vi "Compare Ch with Ch List.vi"(8 "error in (no error)":errorcluster, 10 "Compare List":refnum<class "ChannelVS.lvclass">[](array[class]), 11 "Channel to compare":refnum<class "ChannelVS.lvclass">) -> (0 "error out":errorcluster, 3 "Channel out":refnum<class "ChannelVS.lvclass">)   [LabVIEW 2020, in "Shared Variables CD 2.0 Configuration.lvlib" / "ChannelVS.lvclass"]
uses:
  ChannelVS.lvclass
  ChannelVS.lvclass/ChannelVS.ctl
  built/windows/Channel.lvlibp/Channel.lvclass
  built/windows/Channel.lvlibp/1abvi3w/vi.lib/Utility/Data Type/Type Definitions/Data Type.ctl
  built/windows/Channel.lvlibp/1abvi3w/vi.lib/Utility/Data Type/NI_Data Type.lvlib
  <vilib>/NI VeriStand/Custom Device API/Custom Device Item Ref.ctl
  <vilib>/NI VeriStand/Custom Device API/Custom Device API.lvlib
  C:/Users/Administrator/Desktop/GIT/Shared-Variable-Custom-Device-2.0/Source/built/windows/Channel.lvlibp/Channel.lvclass
  C:/Users/Administrator/Desktop/GIT/Shared-Variable-Custom-Device-2.0/Source/Shared Variables CD 2.0/Configuration/Support/ChannelVS/ChannelVS.lvclass
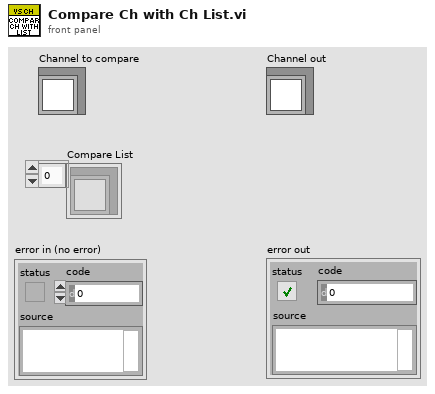
[diagram p1: front panel]
types:
  T1 = typedef "Custom Device API.lvlib/Custom Device Item Ref.ctl" = u64
  T2 = typedef "Channel.lvlibp/NI_Data Type.lvlib/Data Type.ctl" = enum8{"Invalid Type", "Void", "I8", "I16", "I32", "I64", "U8", "U16", "U32", "U64", "Single Float", "Double Float", "Extended Float", "Single Complex", "Double Complex", "Extended Complex", "Enum U8", "Enum U16", "Enum U32", "Enum U64", "Single Float With Unit", "Double Float With Unit", "Extended Float With Unit", "Single Complex with Unit", "Double Complex with Unit", "Extended Complex with Unit", "Boolean", "String", "Path", "Picture", "Tag", "Array", "Cluster", "Variant", "LV Variant", "Waveform", "Timestamp", "Digital Waveform", "Digital Data", "ExpressData", "Refnum", "External Data", "VI", "Poly VI", "LabVIEW Class Instance", "Fixed Point", "Set Collection", "Map Collection"}
  T3 = cluster{"Name":string, "URL":string, "DataType":T2}
  T4 = cluster{"Name":bool, "URL":bool, "DataType":bool}
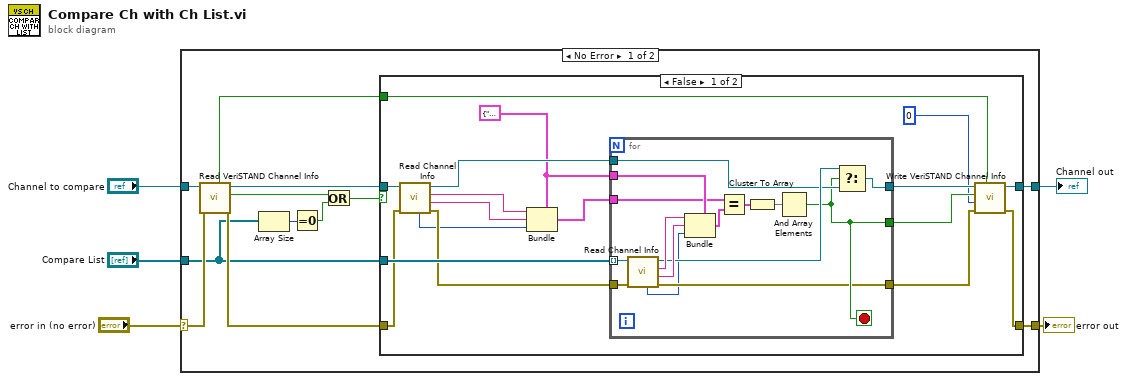
[diagram p0: block diagram]
diagram:
  n1 = case shown="No Error" "error in (no error)" {
    selector: "error in (no error)" -> [w13 w53]
    tunnel: "Compare List" -> [w10 _]
    tunnel: [w17 w52] -> w4
    tunnel: "Channel to compare" -> [w16 w52]
    tunnel: [w11 w53] -> w1
    frame No Error {
      n2 = call "Read VeriSTAND Channel Info.vi"("error in (no error)"=w13, "ChannelVS in"=w16) -> ("error out"=w12:errorcluster, "Exist in VeriSTAND"=w14:bool, "ChannelVS out"=w15:refnum<class "ChannelVS.lvclass">, "Supported in CD"=w6:bool)  [unwired: 5 in, 1 out]
      n3 = Array Size(array=w10) -> (size(s)=w8:i32)
      n4 = Equal To 0?(x=w8) -> (x = 0?=w7:bool)
      n5 = Or(x=w14, y=w7) -> (x .or. y?=w9:bool)
      n6 = case shown="False" w9 {
        tunnel: w10 -> [w34 _]
        tunnel: [w30 w51] -> w17
        tunnel: w15 -> [w27 w51]
        tunnel: w12 -> [w26 w50]
        tunnel: [w23 w50] -> w11
        tunnel: w6 -> [w18 _]
        frame False {
          w31 = T3 {"Name"="", "URL"="", "DataType"=enum."Invalid Type"} ("cluster")
          n7 = call "Read Channel Info.vi"("error in (no error)"=w26, "Channel in"=w27) -> ("error out"=w25:errorcluster, "URL"=w20:string, "Name"=w21:string, "Channel out"=w32:refnum<class "ChannelVS.lvclass">, "DataType"=w19:T2)  [unwired: 4 in, 1 out]
          n8 = Bundle(cluster=w31, "Name"=w21, "URL"=w20, "DataType"=w19) -> (w33:T3)
          n9 = for {
            tunnel: w34 -> [w49] mode=indexing
            tunnel: w33 -> [w44]
            tunnel: w31 -> [w46]
            tunnel: w32 -> [w40]
            tunnel: [w39] -> w28
            tunnel: [w38] -> w29
            tunnel: w25 -> [w37]
            tunnel: [w36] -> w24
            stop <- w38 stop-if-true
            n10 = call "Read Channel Info.vi"("error in (no error)"=w37, "Channel in"=w49) -> ("error out"=w36:errorcluster, "URL"=w47:string, "Name"=w48:string, "Channel out"=w41:refnum<class "ChannelVS.lvclass">, "DataType"=w35:T2)  [unwired: 4 in, 1 out]
            n11 = Bundle(cluster=w46, "Name"=w48, "URL"=w47, "DataType"=w35) -> (w45:T3)
            n12 = Equal?(x=w44, y=w45) -> (x = y?=w43:T4)
            n13 = Cluster To Array(cluster=w43) -> (array=w42:bool[])
            n14 = And Array Elements(Boolean array=w42) -> (logical AND=w38:bool)
            n15 = Select(t=w41, s=w38, f=w40) -> (s? t:f=w39:refnum<class "ChannelVS.lvclass">)
          }
          n16 = call "Write VeriSTAND Channel Info.vi"("Supported in CD"=w18, "error in (no error)"=w24, "VeriSTAND Reference"=T1 0, "Exist in VeriSTAND"=w29, "ChannelVS in"=w28) -> ("error out"=w23:errorcluster, "ChannelVS out"=w30:refnum<class "ChannelVS.lvclass">)  [unwired: 5 in]
        }
        frame True {
        }
      }
    }
    frame Error {
    }
  }
  "Channel out" <- w4
  "error out" <- w1
